vi "Test_Barometer.vi"() -> ()   [LabVIEW 2014]
uses:
  <userlib>/UCSD Robotics Lab/Robotics-Cape/LV/libroboticscape.lvlib
  <vilib>/ptbypt/NI_PtbyPt.lvlib
panel:
  out "Timing Block":T1 {"Actual Hz" format="%#_3g"; "Dt" format="%#_4g"; "Average Hz" format="%#_4g"}
  out "Barometer Output":T2 {"Filtered Altitude (m)" format="%0.2f"}
  out "Iteration counter":i32
  out "State":T3(ring)
  in  "stop":bool
  # "Always stop the VI using the rectangular STOP button above, never with the round stopsign (Abort)"
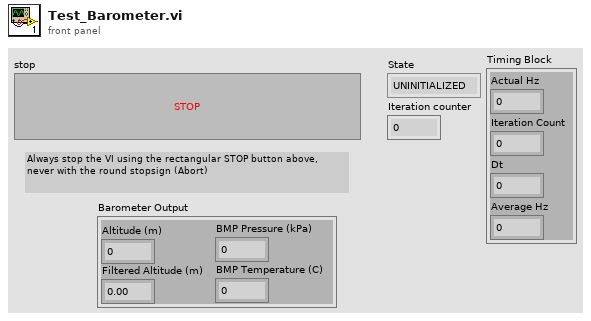
[diagram p1: front panel]
types:
  T1 = cluster{"Actual Hz":dbl, "Iteration Count":dbl, "Dt":dbl, "Average Hz":dbl}
  T2 = cluster{"Altitude (m)":sgl, "Filtered Altitude (m)":dbl, "BMP Pressure (kPa)":sgl, "BMP Temperature (C)":sgl}
  T3 = enum16{"UNINITIALIZED", "RUNNING", "PAUSED", "EXITING"}
  T4 = enum16{"UNINITIALIZED", "RUNING", "PAUSED", "EXITING"}
  T5 = enum32{"Lowpass", "Highpass", "Bandpass", "Bandstop"}
  T6 = cluster{"function return":sgl, "Filtered x":dbl, sgl, "function return":sgl}
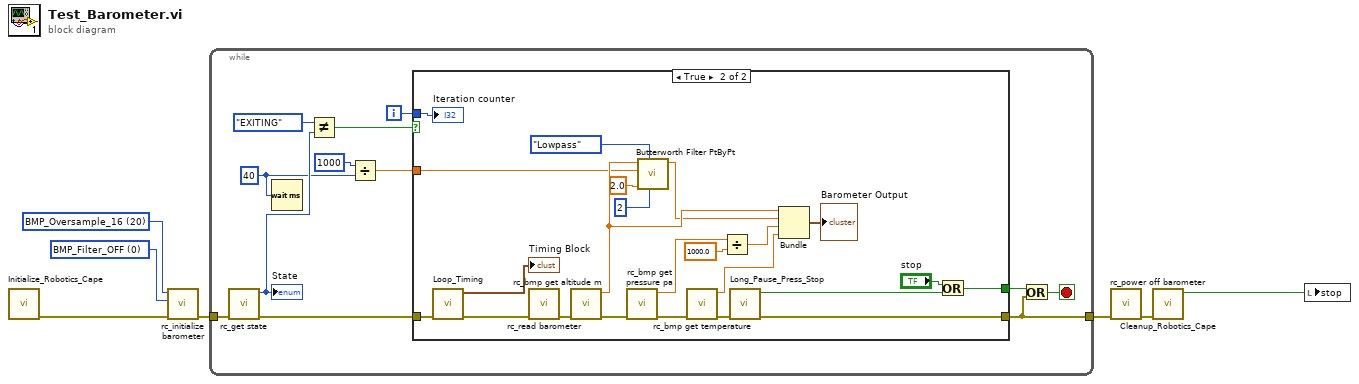
[diagram p0: block diagram]
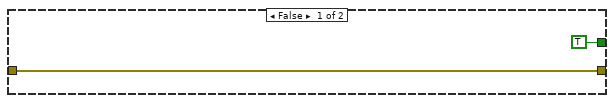
[diagram p2: hidden frame]
diagram:
  w1 = u16 0 items=["BMP_Filter_OFF"=0, "BMP_Filter_2"=4, "BMP_Filter_4"=8, "BMP_Filter_8"=12, "BMP_Filter_16"=16] ("BMP_Filter")
  w2 = u16 20 items=["BMP_Oversample_1"=4, "BMP_Oversample_2"=8, "BMP_Oversample_4"=12, "BMP_Oversample_8"=16, "BMP_Oversample_16"=20] ("BMP_Oversample")
  n1 = call "Initialize_Robotics_Cape.vi"() -> ("error out"=w4:errorcluster)  [unwired: 11 in]
  n2 = call <userlib>:"rc_initialize barometer.vi"("error in (no error)"=w4, "filter"=w1, "oversample"=w2) -> ("error out"=w3:errorcluster)  [unwired: 7 in, 1 out]
  n3 = while {
    tunnel: w3 -> [w18]
    tunnel: [w12] -> w6
    i -> [w17]
    stop <- w19 stop-if-true
    w10 = u32 40 ("milliseconds to wait")
    n4 = call <userlib>:"rc_get state.vi"("error in (no error)"=w18) -> ("error out"=w13:errorcluster, "function return"=w15:u32)  [unwired: 9 in]
    "State" <- w15
    n5 = Wait (ms)(milliseconds to wait=w10) -> ()  [unwired: 1 out]
    n6 = Not Equal?(x=T4."EXITING" ("State 2"), y=w15) -> (x != y?=w14:bool)
    n7 = Divide(x=u32 1000, y=w10) -> (x/y=w8:dbl)
    n8 = case shown="True" w14 {
      tunnel: w17 -> [_ w44]
      tunnel: w13 -> [w21 w33]
      tunnel: [w21 w26] -> w12
      tunnel: [TRUE ("stop") w23] -> w11
      tunnel: w8 -> [_ w22]
      frame False {
      }
      frame True {
        n9 = call "Loop_Timing.vi"("error in"=w33) -> ("error out"=w32:errorcluster, "Timing Block"=→"Timing Block":T1)  [unwired: 9 in]
        n10 = call <userlib>:"rc_read barometer.vi"("error in (no error)"=w32) -> ("error out"=w40:errorcluster)  [unwired: 9 in, 1 out]
        n11 = call <userlib>:"rc_bmp get altitude m.vi"("error in (no error)"=w40) -> ("error out"=w39:errorcluster, "function return"=w37:sgl)  [unwired: 9 in]
        n12 = call <userlib>:"rc_bmp get pressure pa.vi"("error in (no error)"=w39) -> ("error out"=w38:errorcluster, "function return"=w30:sgl)  [unwired: 9 in]
        n13 = call <vilib>:"Butterworth Filter PtByPt.vi"("order"=2, "filter type"=T5."Lowpass", "low cutoff freq: fl"=2.0, "sampling freq: fs"=w22, "x"=w37) -> ("Filtered x"=w36:dbl)  [unwired: 4 in, 1 out]
        n14 = call <userlib>:"rc_bmp get temperature.vi"("error in (no error)"=w38) -> ("error out"=w27:errorcluster, "function return"=w35:sgl)  [unwired: 9 in]
        n15 = Divide(x=w30, y=sgl 1000.0) -> (x/y=w29:sgl)
        n16 = call "Long_Pause_Press_Stop.vi"("error in (no error)"=w27) -> ("error out"=w26:errorcluster, "Stop"=w25:bool)  [unwired: 9 in]
        n17 = Bundle("function return"=w37, "Filtered x"=w36, w29, "function return"=w35) -> (→"Barometer Output":T6)  [unwired: 1 in]
        n18 = Or(x="stop", y=w25) -> (x .or. y?=w23:bool)
        "Iteration counter" <- w44
      }
    }
    n19 = Or(x=w11, y=w12) -> (x .or. y?=w19:bool)
  }
  n20 = call <userlib>:"rc_power off barometer.vi"("error in (no error)"=w6) -> ("error out"=w5:errorcluster)  [unwired: 9 in, 1 out]
  n21 = call "Cleanup_Robotics_Cape.vi"("error in (no error)"=w5) -> ("Stop Local Variabl"=w7:bool)  [unwired: 9 in, 1 out]
  n22 = local write "stop"(w7) -> ()
